vi "Iint.vi"(1 "T":dbl, 2 "ns":dbl, 3 "Rp":dbl, 4 "a":dbl=1.3, 5 "Rs":dbl, 6 "Isc":dbl, 7 "I0":dbl, 8 "Ipv":dbl) -> (0 "Iint":dbl)   [LabVIEW 2016]
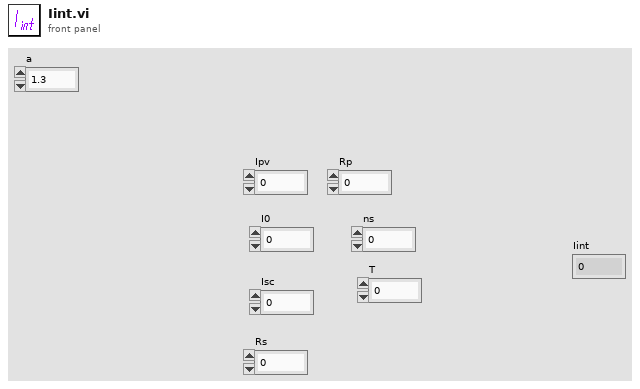
[diagram p1: front panel]
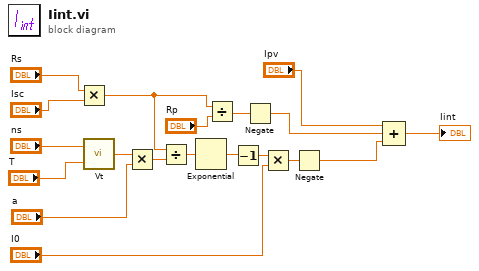
[diagram p0: block diagram]
diagram:
  n1 = Multiply(x="Rs", y="Isc") -> (x*y=w7:dbl)
  n2 = call "Vt.vi"("T"="T", "ns"="ns") -> ("Vt"=w15:dbl)
  n3 = Multiply(x=w15, y="a") -> (x*y=w13:dbl)
  n4 = Divide(x=w7, y=w13) -> (x/y=w12:dbl)
  n5 = Exponential(1:w12) -> (0:w11:dbl)
  n6 = Divide(x=w7, y="Rp") -> (x/y=w3:dbl)
  n7 = Decrement(x=w11) -> (x-1=w10:dbl)
  n8 = Negate(x=w3) -> (-x=w2:dbl)
  n9 = Multiply(x=w10, y="I0") -> (x*y=w4:dbl)
  n10 = Negate(x=w4) -> (-x=w1:dbl)
  n11 = Compound Arithmetic op=ADD("Ipv", w2, w1) -> (→"Iint":dbl)
